vi "NSSGP.vi"() -> ()   [LabVIEW 2020]
uses:
  Data Cluster.ctl
panel:
  in  "Tab Control":enum32{"Pressure", "Permeance"}(tab)
  out "Feed Pressure [Pa]":dbl format="%#.2g"
  out "Feed Pressure [Pa]":cluster{dbl[], dbl[]}(graph)
  out "Permeate Pressure [Pa]":dbl format="%#.2g"
  out "Permeate Pressure [Pa]":dbl format="%#.2g"
  out "Time [s]":dbl format="%#.2g"
  out "Feed Pressure [Pa]":dbl format="%#.2g"
  out "Permeate Pressure [Pa]":cluster{dbl[], dbl[]}(graph)
  in  "Logging?":bool
  in  "stop":bool
  # "Non-stationary Single Gas Permeation (Feed-side Relaxation)"
  # "Version: 1.0"
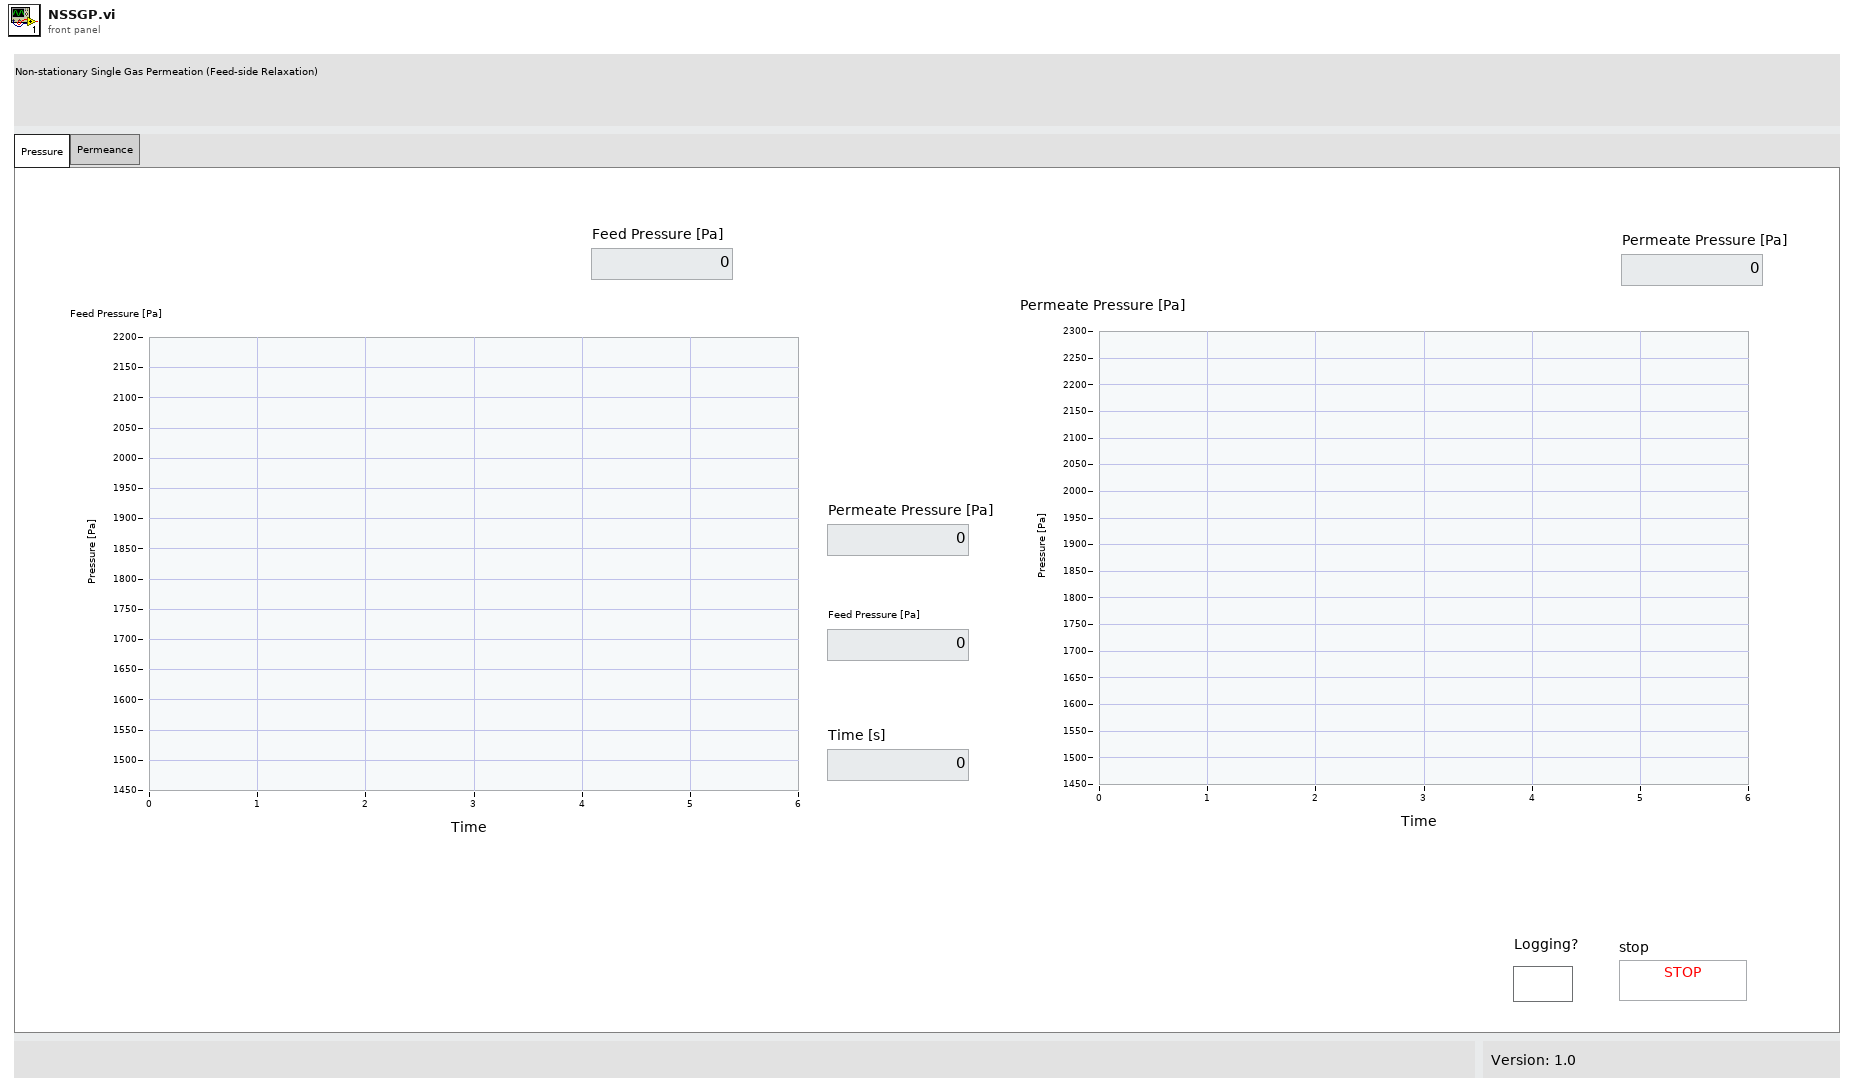
[diagram p1: front panel]
types:
  T1 = typedef "Data Cluster.ctl" = cluster{"Time Array":dbl[], "Feed P Array":dbl[], "Permeate P Array":dbl[]}
  T2 = enum16{"open", "open or create", "create or replace", "create", "open (read-only)"}
  T3 = cluster{"Time Array":dbl[], "Feed P Array":dbl[]}
  T4 = cluster{"Time Array":dbl[], "Permeate P Array":dbl[]}
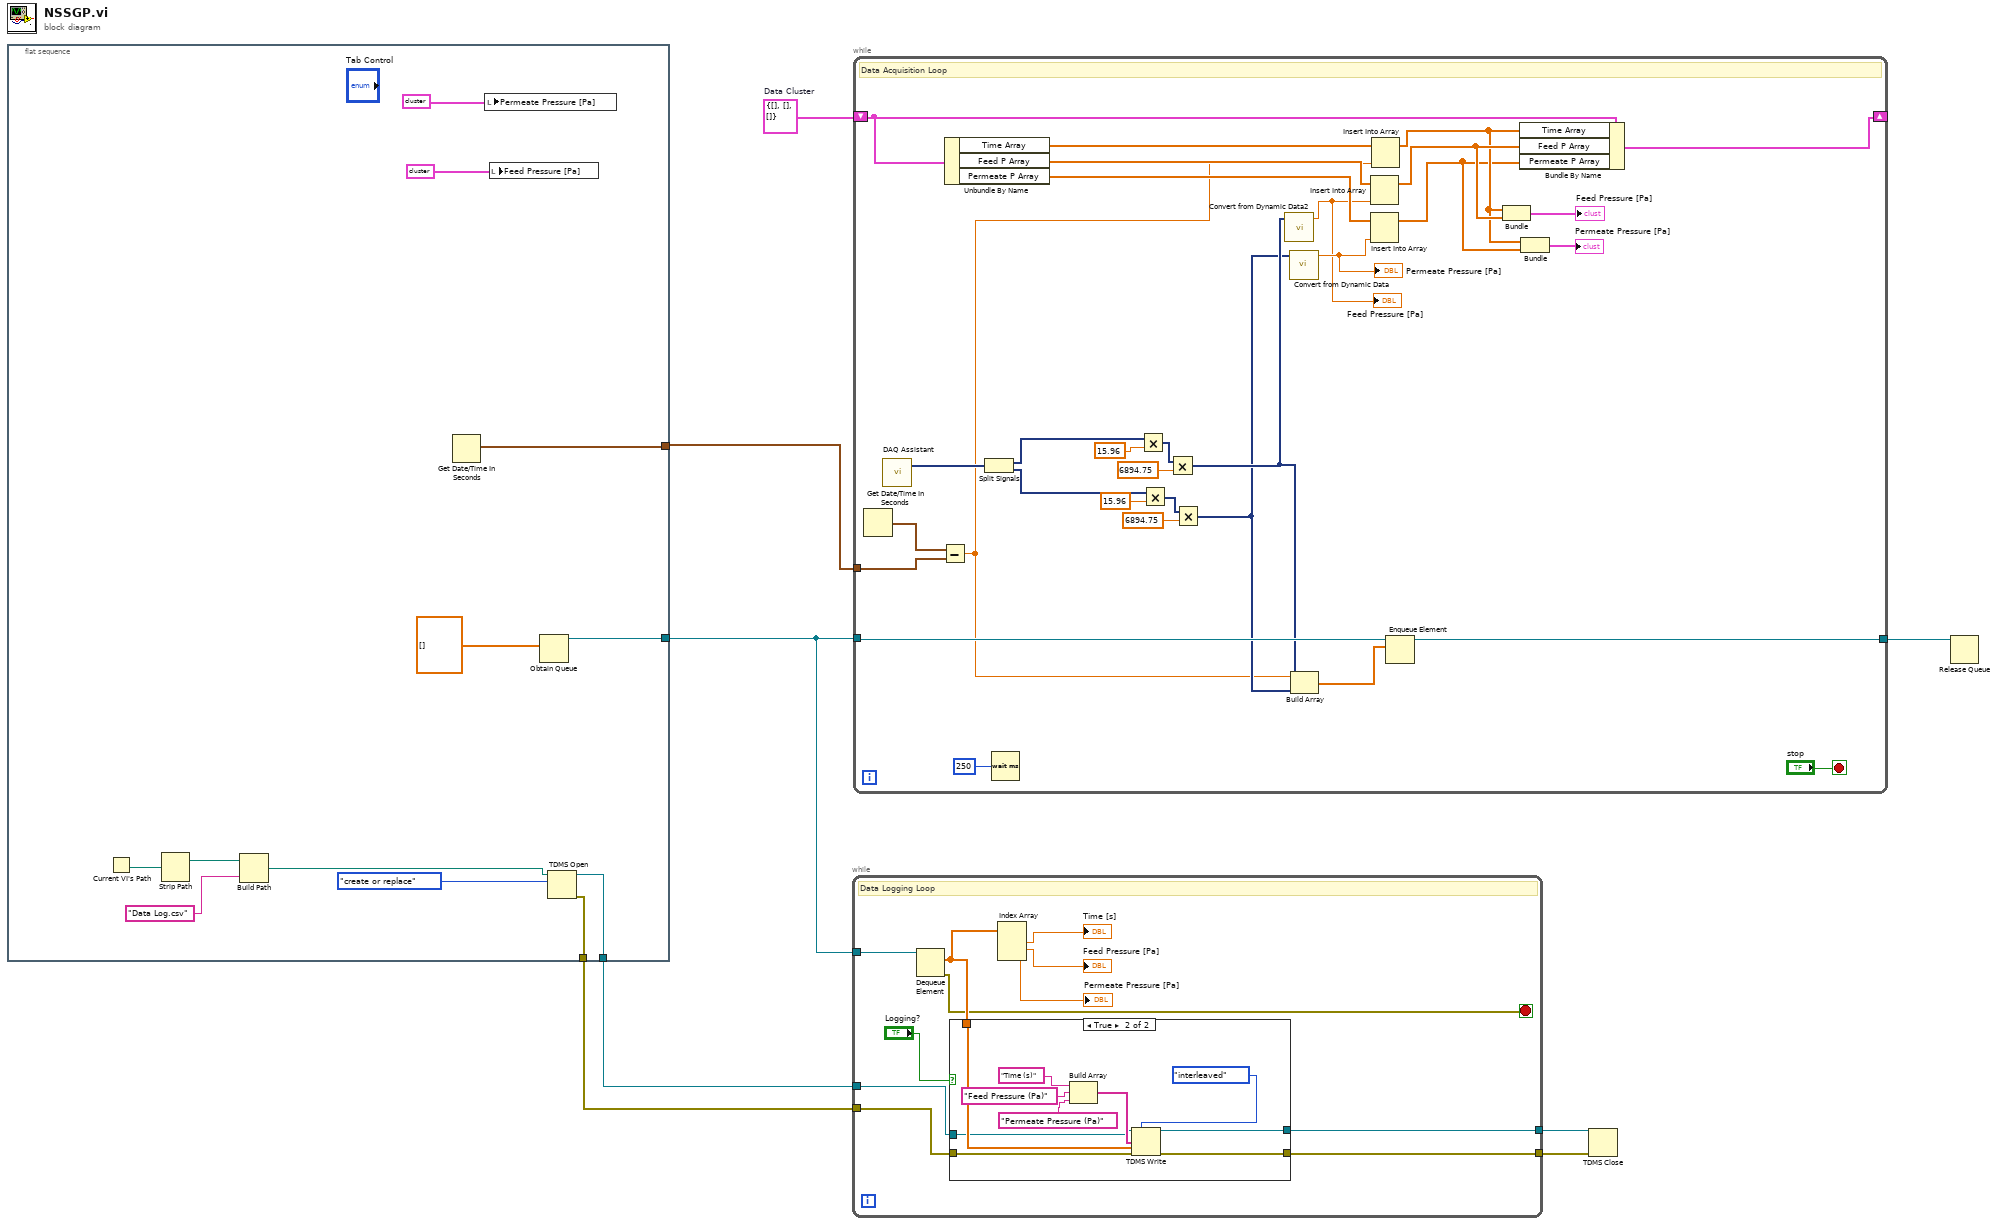
[diagram p0: block diagram]
diagram:
  w1 = T1 {"Time Array"=[], "Feed P Array"=[], "Permeate P Array"=[]}  # Data Cluster
  n1 = flat-sequence {
    tunnel: [w18] -> w5
    tunnel: [w16] -> w4
    tunnel: [w14] -> w3
    tunnel: [w13] -> w2
    frame #0 {
      n2 = Current VI's Path() -> (path=w12:path)
      n3 = Strip Path(path=w12) -> (stripped path=w11:path)  [unwired: 1 out]
      n4 = Build Path(base path=w11, name or relative path="Data Log.csv") -> (appended path=w10:path)
      n5 = Get Date/Time In Seconds() -> (seconds since 1Jan1904=w18:timestamp)
      n6 = local write "Permeate Pressure [Pa]"(cluster{dbl[], dbl[]} {array[1217 elements], array[1217 elements]} ("XY Graph 2")) -> ()
      n7 = local write "Feed Pressure [Pa]"(cluster{dbl[], dbl[]} {array[1217 elements], array[1217 elements]} ("XY Graph")) -> ()
      n8 = Obtain Queue(element data type=dbl[] []) -> (queue out=w16:refnum<queue>)  [unwired: 4 in, 2 out]
      n9 = TDMS Open(10:T2."create or replace" ("operation (0:open)"), 11:w10) -> (0:w14:errorcluster, 3:w13:refnum<k34>)  [unwired: 5 in]
    }
  }
  n10 = while {
    tunnel: w4 -> [w31]
    tunnel: [w27] -> w7
    tunnel: [w22] -> w6
    tunnel: w2 -> [w25]
    tunnel: w3 -> [w26]
    stop <- w21 stop-if-true
    # "Data Logging Loop"
    n11 = Dequeue Element(queue=w31) -> (element=w23:dbl[], error out=w21:errorcluster)  [unwired: 2 in, 2 out]
    n12 = case shown="True" "Logging?" {
      tunnel: [w33 w34] -> w27
      tunnel: [w32 w38] -> w22
      tunnel: w26 -> [w32 w37]
      tunnel: w25 -> [w33 w35]
      tunnel: w23 -> [_ w36]
      frame False {
      }
      frame True {
        n13 = Build Array("Time (s)", "Feed Pressure (Pa)", "Permeate Pressure (Pa)") -> (w43:string[])
        n14 = TDMS Write(0:w35, 1:enum16{"decimated", "interleaved"}."interleaved" ("data layout (0:decimated)"), 7:w43, 9:w36, 11:w37) -> (4:w34:refnum<k34>, 15:w38:errorcluster)  [unwired: 1 in, 2 out]
      }
    }
    n15 = Index Array(array=w23) -> (element #1=→"Time [s]":dbl, element #2=→"Feed Pressure [Pa]":dbl, element #3=→"Permeate Pressure [Pa]":dbl)  [unwired: 3 in]
  }
  n16 = while {
    tunnel: w4 -> [w74]
    tunnel: [w72] -> w8
    tunnel: w5 -> [w69]
    shift-right: [w49] -> _
    shift-left: w1 -> [w50]
    stop <- "stop" stop-if-true
    # "Data Acquisition Loop"
    n17 = Get Date/Time In Seconds() -> (seconds since 1Jan1904=w70:timestamp)
    n18 = call "DAQ Assistant"() -> ("data"=w68:dynamicdata)  [unwired: 17 in, 2 out]
    n19 = Subtract(x=w70, y=w69) -> (x-y=w53:dbl)
    n20 = Unbundle By Name(w50) -> ("Time Array"=w56:dbl[], "Feed P Array"=w55:dbl[], "Permeate P Array"=w54:dbl[])
    n21 = Split Signals(w68) -> (w64:dynamicdata, w60:dynamicdata)  [unwired: 2 in]
    n22 = Wait (ms)(milliseconds to wait=u32 250 ("y")) -> ()  [unwired: 1 out]
    n23 = Multiply(x=w64, y=15.96) -> (x*y=w66:dynamicdata)
    n24 = Multiply(x=w60, y=15.96) -> (x*y=w62:dynamicdata)
    n25 = Multiply(x=w66, y=6894.75) -> (x*y=w58:dynamicdata)
    n26 = Multiply(x=w62, y=6894.75) -> (x*y=w57:dynamicdata)
    n27 = call "Convert from Dynamic Data2"("Dynamic Data Type"=w58) -> ("Scalar"=w51:dbl)  [unwired: 3 in]
    "Feed Pressure [Pa]" <- w51
    n28 = call "Convert from Dynamic Data"("Dynamic Data Type"=w57) -> ("Scalar"=w52:dbl)  [unwired: 3 in]
    "Permeate Pressure [Pa]" <- w52
    n29 = Build Array(w53, w58, w57) -> (w73:dbl[])
    n30 = Insert Into Array(array=w55, new element=w51) -> (w48:dbl[])  [unwired: 1 in]
    n31 = Insert Into Array(array=w54, new element=w52) -> (w45:dbl[])  [unwired: 1 in]
    n32 = Insert Into Array(array=w56, new element=w53) -> (w46:dbl[])  [unwired: 1 in]
    n33 = Enqueue Element(queue=w74, element=w73) -> (queue out=w72:refnum<queue>)  [unwired: 2 in, 2 out]
    n34 = Bundle("Time Array"=w46, "Feed P Array"=w48) -> (→"Feed Pressure [Pa]":T3)  [unwired: 1 in]
    n35 = Bundle By Name(cluster=w50, "Time Array"=w46, "Feed P Array"=w48, "Permeate P Array"=w45) -> (w49:T1)
    n36 = Bundle("Time Array"=w46, "Permeate P Array"=w45) -> (→"Permeate Pressure [Pa]":T4)  [unwired: 1 in]
  }
  n37 = TDMS Close(8:w6, 11:w7) -> ()  [unwired: 2 out]
  n38 = Release Queue(queue=w8) -> ()  [unwired: 2 in, 3 out]
